vi "niRFUtil FWK Check Driver Version.vi"(8 "error in (no error)":errorcluster, 11 "Instr Info":T1={"Check Version?"=TRUE, "Instr type"=enum."RFInstr Agn", "Major Version"="1", "Minor Version"="1", "Registry Key"=[], "Product Name"="NI"}) -> (0 "error out":errorcluster)   [LabVIEW 2015, in "niRFUtil.lvlib"]
uses:
  niRFUtil.lvlib
  Includes/niRFUtil INC FWK Instrument Version Info.ctl
  Includes/niRFUtil INC FWK Class Types.ctl
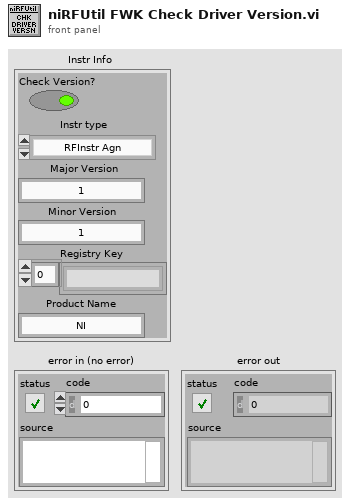
[diagram p1: front panel]
types:
  T1 = typedef "niRFUtil.lvlib/niRFUtil INC FWK Instrument Version Info.ctl" = cluster{"Check Version?":bool, "Instr type":T2, "Major Version":string, "Minor Version":string, "Registry Key":string[], "Product Name":string}
  T2 = typedef "niRFUtil.lvlib/niRFUtil INC FWK Class Types.ctl" = enum16{"RFInstr Agn", "RFSAInstr", "DCPowerInstr"}
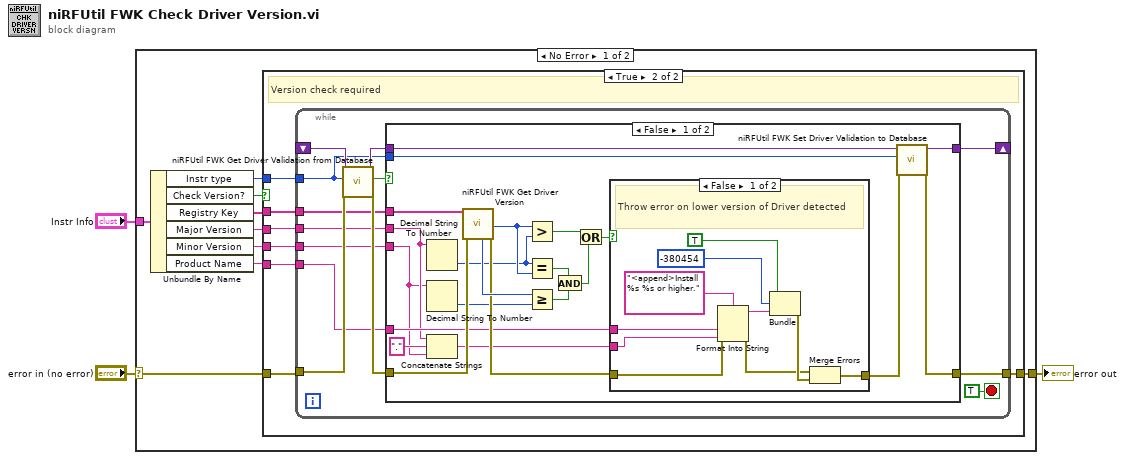
[diagram p0: block diagram]
diagram:
  n1 = case shown="No Error" "error in (no error)" {
    selector: "error in (no error)" -> [w12 w69]
    tunnel: [w11 w69] -> w3
    tunnel: "Instr Info" -> [w10 _]
    frame No Error {
      n2 = Unbundle By Name(w10) -> ("Instr type"=w6:T2, "Check Version?"=w5:bool, "Registry Key"=w7:string[], "Major Version"=w9:string, "Minor Version"=w8:string, "Product Name"=w4:string)
      n3 = case shown="True" w5 {
        tunnel: w12 -> [w13 w20]
        tunnel: [w13 w17] -> w11
        tunnel: w9 -> [_ w19]
        tunnel: w8 -> [_ w18]
        tunnel: w6 -> [_ w16]
        tunnel: w7 -> [_ w15]
        tunnel: w4 -> [_ w14]
        frame False {
          # "Version check not required"
        }
        frame True {
          # "Version check required"
          n4 = while {
            tunnel: w20 -> [w33]
            tunnel: w19 -> [w23]
            tunnel: w18 -> [w22]
            tunnel: [w32] -> w17
            shift-right: [w29] -> _
            shift-left: _ -> [w30]
            tunnel: w16 -> [w25]
            tunnel: w15 -> [w24]
            tunnel: w14 -> [w21]
            stop <- TRUE stop-if-true
            n5 = call "niRFUtil FWK Get Driver Validation from Database.vi"("error in (no error)"=w33, "Loaded Driver Type"=w25, "Driver Validation Database In"=w30) -> ("error out"=w28:errorcluster, "Valid Driver?"=w26:bool, "Driver Validation Database Out"=w27:variant)  [unwired: 6 in]
            n6 = case shown="False" w26 {
              tunnel: [w51 w67] -> w32
              tunnel: [w50 w68] -> w29
              tunnel: w28 -> [w49 w67]
              tunnel: w27 -> [w48 w68]
              tunnel: w25 -> [w42 _]
              tunnel: w21 -> [w41 _]
              tunnel: w24 -> [w40 _]
              tunnel: w23 -> [w36 _]
              tunnel: w22 -> [w35 _]
              frame False {
                n7 = Decimal String To Number(string=w36) -> (number=w39:i32)  [unwired: 2 in, 1 out]
                n8 = Decimal String To Number(string=w35) -> (number=w38:i32)  [unwired: 2 in, 1 out]
                n9 = Concatenate Strings(w36, "." ("string"), w35) -> (w34:string)
                n10 = call "niRFUtil FWK Get Driver Version.vi"("error in (no error)"=w49, "Registry Key"=w40) -> ("error out"=w52:errorcluster, "Major Version"=w55:i32, "Minor Version"=w54:i32)  [unwired: 5 in, 2 out]
                n11 = Greater?(x=w55, y=w39) -> (0:w45:bool)
                n12 = Equal?(x=w39, y=w55) -> (x = y?=w47:bool)
                n13 = Greater Or Equal?(x=w54, y=w38) -> (x >= y?=w46:bool)
                n14 = And(x=w47, y=w46) -> (x .and. y?=w44:bool)
                n15 = Or(x=w45, y=w44) -> (x .or. y?=w43:bool)
                n16 = case shown="False" w43 {
                  tunnel: w52 -> [w59 w66]
                  tunnel: w34 -> [w57 _]
                  tunnel: [w58 w66] -> w53
                  tunnel: w41 -> [w56 _]
                  frame False {
                    # "Throw error on lower version of Driver detected"
                    n17 = Format Into String(format string="<append>Install %s %s or higher." ("error message (\"\")"), error in=w59, w56, w57) -> (resulting string=w64:string, error out=w61:errorcluster)  [unwired: 1 in]
                    n18 = Bundle(TRUE, "error code (0)"=-380454, w64) -> (w62:cluster{bool, "error code (0)":i32, string})  [unwired: 1 in]
                    n19 = Merge Errors(w61, w62) -> (w58:errorcluster)
                  }
                  frame True {
                    # "Installed Driver matches the minimum requirement"
                  }
                }
                n20 = call "niRFUtil FWK Set Driver Validation to Database.vi"("error in (no error)"=w53, "Loaded Driver Type"=w42, "Driver Validation Database In"=w48) -> ("error out"=w51:errorcluster, "Driver Validation Database Out"=w50:variant)  [unwired: 7 in]
              }
              frame True {
                # "Doesn't require any driver validation since it was already performed on the \nprevious calls"
              }
            }
          }
        }
      }
    }
    frame Error {
    }
  }
  "error out" <- w3
